vi "F_a_2.vi"   [LabVIEW 2014]
uses:
  <vilib>/imath/engines/lvmath2/RunTimeEngine/Managers/WorkSpace/UID Generator.vi
  <vilib>/imath/engines/lvmath2/RunTimeEngine/RangeToken/NIMS_Range_R2 - Integer.vi
  <instcachedir>/0/NIMS_Range_R2 - Integer_2D1304BAF97744E0A293025746CBADFC.lvgen/NIMS_Range_R2 - Integer_2D1304BAF97744E0A293025746CBADFC_000.vi
  <vilib>/imath/engines/lvmath2/RunTimeEngine/CommandStatement/MC_CommandStatement_break.vi
  <vilib>/imath/engines/lvmath2/RunTimeEngine/VariableToken/NIMS_VariableToken_CondDefinedDefinedByReplace.vi
  <instcachedir>/0/NIMS_VariableToken_CondDefinedDefinedByReplace_D162CFFC24174562A9FEA619A91E1A56.lvgen/NIMS_VariableToken_CondDefinedDefinedByReplace_D162CFFC24174562A9FEA619A91E1A56_002.vi
  <vilib>/imath/engines/lvmath2/RunTimeEngine/BuiltInFunctions/round/NIMS_round(DBL-S).vi
  <vilib>/imath/engines/lvmath2/RunTimeEngine/IndexReplace/NIMS V(S)=S.vi
  <instcachedir>/0/NIMS V(S)=S_2D52C4EC15D8415E870AEE69FB516CCA.lvgen/NIMS V(S)=S_2D52C4EC15D8415E870AEE69FB516CCA_000.vi
  <vilib>/imathl/engines/lvmath/Functions/Error Handling/Create Error.vi
  <vilib>/imath/engines/lvmath2/RunTimeEngine/VariableToken/NIMS_VariableToken_CondDefined.vi
  <instcachedir>/0/NIMS_VariableToken_CondDefined_EE8DD211A89249938CE6537267F5C9B3.lvgen/NIMS_VariableToken_CondDefined_EE8DD211A89249938CE6537267F5C9B3_003.vi
  <vilib>/imath/engines/lvmath2/RunTimeEngine/ArithmeticOperatorToken/NIMS_ArithmeticOperator_plus.vi
  <instcachedir>/0/NIMS_ArithmeticOperator_plus_48D6EAACA5D645B09F7EC9C016C2DEA8.lvgen/NIMS_ArithmeticOperator_plus_48D6EAACA5D645B09F7EC9C016C2DEA8_004.vi
  <vilib>/imath/engines/lvmath2/RunTimeEngine/ErrorHandling/NIMS_Create Error From Enums.vi
  <vilib>/imath/engines/lvmath2/RunTimeEngine/BuiltInFunctions/plot/NIMS_plot(G, Str).vi
  <instcachedir>/0/NIMS_plot(G, Str)_63281ED914EA4C6894EA6911D34D3931.lvgen/NIMS_plot(G, Str)_63281ED914EA4C6894EA6911D34D3931_000.vi
  <vilib>/imath/engines/lvmath2/RunTimeEngine/IndexRead/NIMS V(S).vi
  <instcachedir>/0/NIMS V(S)_0488751826AF41519A22953C041130DC.lvgen/NIMS V(S)_0488751826AF41519A22953C041130DC_000.vi
  <vilib>/imath/engines/lvmath2/RunTimeEngine/RangeToken/NIMS_Range_R3 - Integer.vi
  <instcachedir>/0/NIMS_Range_R3 - Integer_66B9031982364693905FDE422E56E490.lvgen/NIMS_Range_R3 - Integer_66B9031982364693905FDE422E56E490_000.vi
  <instcachedir>/0/NIMS_VariableToken_CondDefined_EE8DD211A89249938CE6537267F5C9B3.lvgen/NIMS_VariableToken_CondDefined_EE8DD211A89249938CE6537267F5C9B3_004.vi
  <vilib>/imath/engines/lvmath2/RunTimeEngine/BuiltInFunctions/fft/NIMS_fft(GV).vi
  <instcachedir>/0/NIMS_fft(GV)_4C6467FC22F84E4BA42517A07EF978B0.lvgen/NIMS_fft(GV)_4C6467FC22F84E4BA42517A07EF978B0_000.vi
  <vilib>/imath/engines/lvmath2/RunTimeEngine/ErrorHandling/NIMS_Error From Error Code.vi
  <vilib>/imath/engines/lvmath2/RunTimeEngine/BuiltInFunctions/abs/NIMS_abs(signed).vi
  <instcachedir>/0/NIMS_abs(signed)_C4FCB8E6058B49B797C7C8D53CA5F6EC.lvgen/NIMS_abs(signed)_C4FCB8E6058B49B797C7C8D53CA5F6EC_006.vi
  <vilib>/imath/engines/lvmath2/RunTimeEngine/BuiltInFunctions/subplot/NIMS_subplot(I32, I32, I32).vi
  <vilib>/imath/engines/lvmath2/RunTimeEngine/BuiltInFunctions/grid/NIMS_grid(Enums).vi
  <vilib>/imath/engines/lvmath2/RunTimeEngine/BuiltInFunctions/pause/NIMS_pause(S).vi
  <vilib>/imath/engines/lvmath2/RunTimeEngine/CommandStatement/NIMS_CommandStatement_MaskErr.vi
  <vilib>/imath/engines/lvmath2/RunTimeEngine/Managers/SymbolTable/Clear UID.vi
  <vilib>/imath/engines/lvmath2/RunTimeEngine/ErrorHandling/NIMS_Finalize Error.vi
  <vilib>/imath/engines/lvmath2/RunTimeEngine/Managers/SymbolTable/NIMS_WorkSpace.lvlib
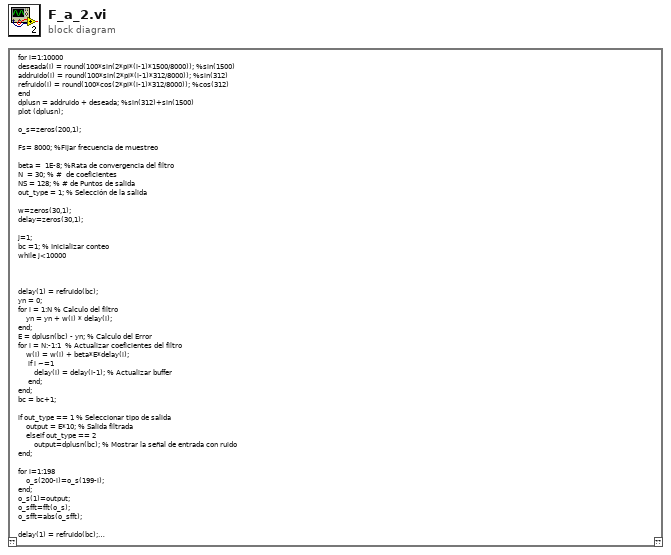
[diagram p0: block diagram]
diagram:
  n1 = mathscript code="for i=1:10000\ndeseada(i) = round(100*sin(2*pi*(i-1)*1500/8000)); %sin(1500)\naddruido(i) = round(100*sin(2*pi*(i-1)*312/8000)); %sin(312)\nrefruido(i) = round(100*cos(2*pi*(i-1)*312/8000)); %cos(312)\nend\ndplusn = addruido + deseada; %sin(312)+sin(1500)\nplot (dplusn);\n\no_s=zeros(200,1);\n\nFs= 8000; %Fijar frecuencia de muestreo\n\nbeta =  1E-8; %Rata de convergencia del filtro\nN  = 30; % #  de coeficientes \nNS = 128; % # de Puntos de salida\nout_type = 1; % Selección de la salida\n\nw=zeros(30,1);\ndelay=zeros(30,1);\n\nj=1;\nbc =1; % Inicializar conteo\nwhile j<10000\n\n\n\ndelay(1) = refruido(bc); \nyn = 0; \nfor i = 1:N % Calculo del filtro\n    yn = yn + w(i) * delay(i); \nend;\nE = dplusn(bc) - yn; % Calculo del Error\nfor i = N:-1:1  % Actualizar coeficientes del filtro\n    w(i) = w(i) + beta*E*delay(i); \n     if i ~=1        \n        delay(i) = delay(i-1); % Actualizar buffer\n     end;\nend;\nbc = bc+1;\n\nif out_type == 1 % Seleccionar tipo de salida\n    output = E*10; % Salida filtrada\n    elseif out_type == 2\n        output=dplusn(bc); % Mostrar la señal de entrada con ruido\nend;\n\nfor i=1:198\n    o_s(200-i)=o_s(199-i);\nend;\no_s(1)=output; \no_sfft=fft(o_s);\no_sfft=abs(o_sfft);\n\ndelay(1) = refruido(bc); \nsubplot (2,1,1),plot (o_s);\ngrid on;\nsubplot (2,1,2),plot (o_sfft);\ngrid on;\nj=j+1;\npause(0.01);\nend;"() -> ()  [unwired: 1 in, 1 out]
